vi "Initialize.vi"(8 "error in (no error)":errorcluster, 9 "ID Query":bool, 10 "Reset":bool, 11 "Yokogawa WT1600 in":refnum<class "Yokogawa WT1600.lvclass">) -> (0 "error out":errorcluster, 2 "VISA resource name":refnum<visa-resource-name>, 3 "Yokogawa WT1600 out":refnum<class "Yokogawa WT1600.lvclass">)   [LabVIEW 2014, in "Generic Power Analyzer.lvlib" / "Yokogawa WT1600.lvlib" / "Yokogawa WT1600.lvclass"]
uses:
  Yokogawa WT1600.lvclass
  Generic Power Analyzer/Generic Power Analyzer.lvclass
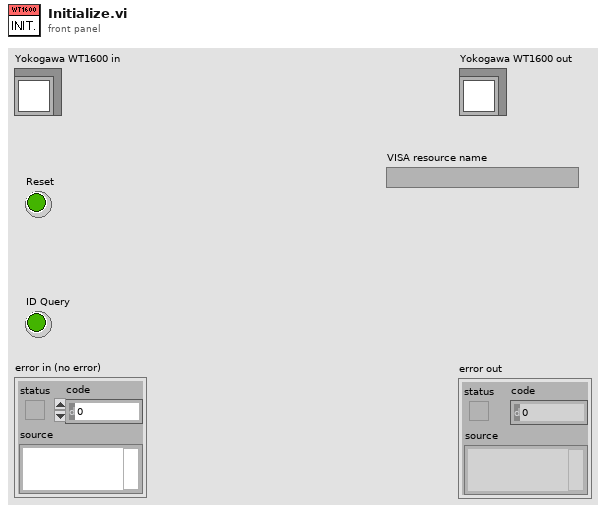
[diagram p1: front panel]
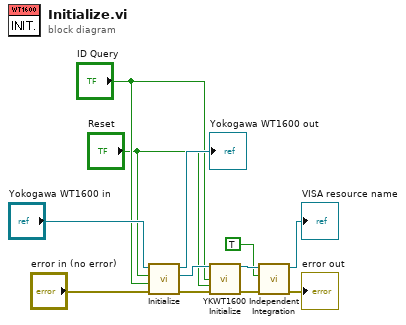
[diagram p0: block diagram]
diagram:
  n1 = call-parent "Initialize.vi"("error in (no error)"="error in (no error)", "ID Query"="ID Query", "Reset"="Reset", "Generic Power Analyzer in"="Yokogawa WT1600 in") -> ("error out"=w4:errorcluster, "VISA resource name"=w7:refnum<visa-resource-name>, "Generic Power Analyzer out"=→"Yokogawa WT1600 out":refnum<class "Yokogawa WT1600.lvclass">)  [unwired: 5 in]
  n2 = call <instrlib>:"YKWT1600 Initialize.vi"("VISA session (for class)"=w7, "ID Query (T: Check)"="ID Query", "Reset (T: Reset)"="Reset", "error in (no error)"=w4) -> ("VISA session"=w12:refnum<visa-resource-name>, "error out"=w9:errorcluster)  [unwired: 10 in]
  n3 = call "Independent Integration.vi"("error in"=w9, "ON/OFF"=TRUE, "VISA resource name"=w12) -> ("error out"=→"error out":errorcluster, "VISA resource name out"=→"VISA resource name":refnum<visa-resource-name>)  [unwired: 7 in]
